vi "PWM Set Pulse.vi"(9 "pPulse":u16, 10 "ChannelMask":u8, 11 "DevIndex":i32) -> (1 "pPulse out":u16, 3 "function return":i32)   [LabVIEW 2010, in "usb2pwm.lvlib"]
doc: "int WINAPI PWM_SetPulse(int DevIndex,unsigned char ChannelMask,unsigned short *pPulse);"
uses:
  usb2pwm.lvlib
  USB2XXX.dll
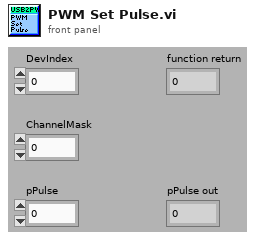
[diagram p1: front panel]
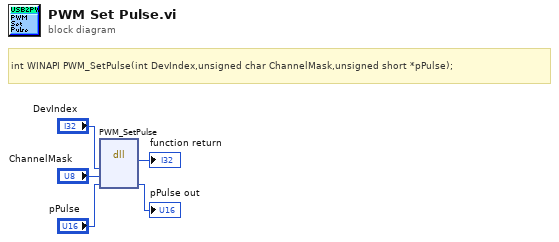
[diagram p0: block diagram]
diagram:
  # "int WINAPI PWM_SetPulse(int DevIndex,unsigned char ChannelMask,unsigned short *pPulse);"
  n1 = dll-call lib="G:/OtherWork/USB2XXX_Example/trunk/Labview/PublicFiles/usb2pwm/USB2XXX.*" fn="PWM_SetPulse"("DevIndex"="DevIndex", "ChannelMask"="ChannelMask", "pPulse"="pPulse") -> (→"function return":i32, "pPulse"=→"pPulse out":u16)  [unwired: 5 in, 2 out]
